vi "脉冲测试脚本.vi"(1 "参数":T1) -> (0 "Script":string)   [LabVIEW 2020]
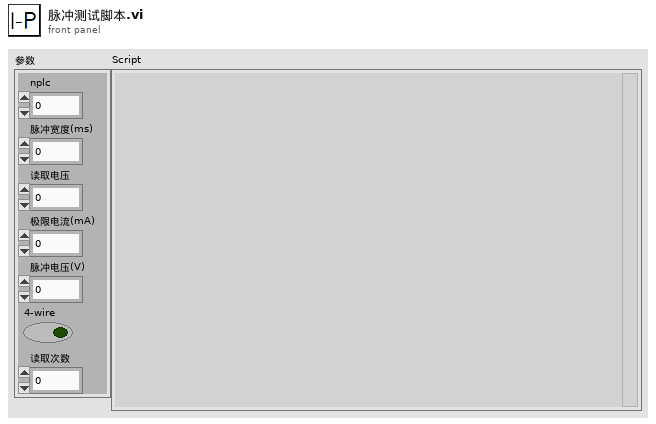
[diagram p1: front panel]
types:
  T1 = cluster{"nplc":dbl, "脉冲宽度(ms)":dbl, "读取电压":dbl, "极限电流(mA)":dbl, "脉冲电压(V)":dbl, "4-wire":bool, "读取次数":dbl}
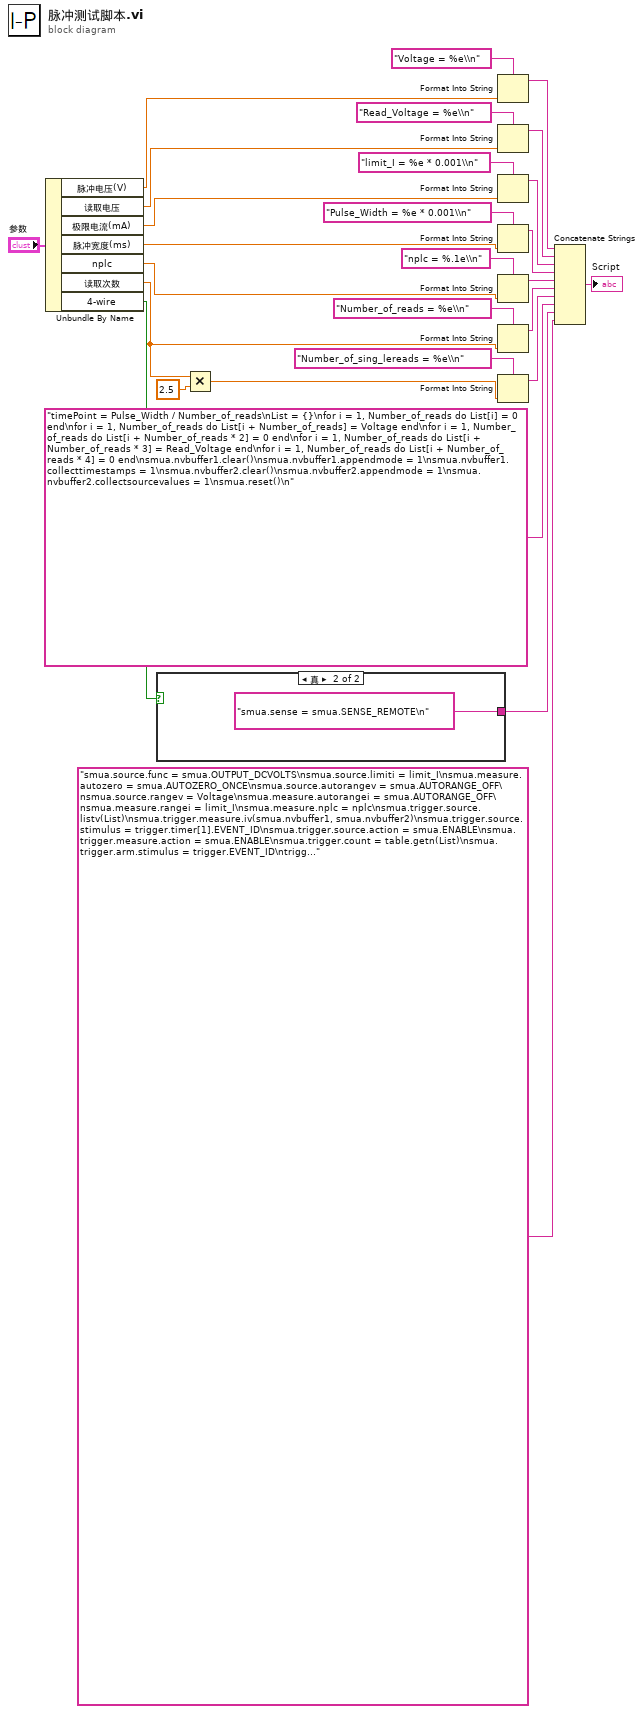
[diagram p0: block diagram]
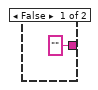
[diagram p2: hidden frame]
diagram:
  n1 = Unbundle By Name("参数") -> ("脉冲电压(V)"=w15:dbl, "读取电压"=w14:dbl, "极限电流(mA)"=w13:dbl, "脉冲宽度(ms)"=w12:dbl, "nplc"=w4:dbl, "读取次数"=w3:dbl, "4-wire"=w8:bool)
  n2 = case shown="真" w8 {
    tunnel: ["" "smua.sense = smua.SENSE_REMOTE\n"] -> w16
    frame False {
    }
    frame True {
    }
  }
  n3 = Multiply(x=w3, y=2.5) -> (x*y=w1:dbl)
  n4 = Format Into String(format string="Voltage = %e\\n" ("格式字符串"), w15) -> (resulting string=w25:string)  [unwired: 2 in, 1 out]
  n5 = Format Into String(format string="Read_Voltage = %e\\n" ("格式字符串"), w14) -> (resulting string=w23:string)  [unwired: 2 in, 1 out]
  n6 = Format Into String(format string="limit_I = %e * 0.001\\n" ("格式字符串"), w13) -> (resulting string=w22:string)  [unwired: 2 in, 1 out]
  n7 = Format Into String(format string="Pulse_Width = %e * 0.001\\n", w12) -> (resulting string=w20:string)  [unwired: 2 in, 1 out]
  n8 = Format Into String(format string="nplc = %.1e\\n", w4) -> (resulting string=w18:string)  [unwired: 2 in, 1 out]
  n9 = Format Into String(format string="Number_of_reads = %e\\n" ("格式字符串"), w3) -> (resulting string=w6:string)  [unwired: 2 in, 1 out]
  n10 = Format Into String(format string="Number_of_sing_lereads = %e\\n" ("格式字符串"), w1) -> (resulting string=w5:string)  [unwired: 2 in, 1 out]
  n11 = Concatenate Strings(w25, w23, w22, w20, w18, w6, w5, "timePoint = Pulse_Width / Number_of_reads\nList = {}\nfor i = 1, Number_of_reads do List[i] = 0 end\nfor i = 1, Number_of_reads do List[i + Number_of_reads] = Voltage end\nfor i = 1, Number_of_reads do List[i + Number_of_reads * 2] = 0 end\nfor i = 1, Number_of_reads do List[i + Number_of_reads * 3] = Read_Voltage end\nfor i = 1, Number_of_reads do List[i + Number_of_reads * 4] = 0 end\nsmua.nvbuffer1.clear()\nsmua.nvbuffer1.appendmode = 1\nsmua.nvbuffer1.collecttimestamps = 1\nsmua.nvbuffer2.clear()\nsmua.nvbuffer2.appendmode = 1\nsmua.nvbuffer2.collectsourcevalues = 1\nsmua.reset()\n", w16, "smua.source.func = smua.OUTPUT_DCVOLTS\nsmua.source.limiti = limit_I\nsmua.measure.autozero = smua.AUTOZERO_ONCE\nsmua.source.autorangev = smua.AUTORANGE_OFF\nsmua.source.rangev = Voltage\nsmua.measure.autorangei = smua.AUTORANGE_OFF\nsmua.measure.rangei = limit_I\nsmua.measure.nplc = nplc\nsmua.trigger.source.listv(List)\nsmua.trigger.measure.iv(smua.nvbuffer1, smua.nvbuffer2)\nsmua.trigger.source.stimulus = trigger.timer[1].EVENT_ID\nsmua.trigger.source.action = smua.ENABLE\nsmua.trigger.measure.action = smua.ENABLE\nsmua.trigger.count = table.getn(List)\nsmua.trigger.arm.stimulus = trigger.EVENT_ID\ntrigger.timer[1].reset()\ntrigger.timer[1].stimulus = smua.trigger.ARMED_EVENT_ID\ntrigger.timer[1].passthrough = false\ntrigger.timer[1].delay = timePoint\ntrigger.timer[1].count = table.getn(List)\nsmua.source.output = smua.OUTPUT_ON\nsmua.trigger.initiate()\ndelay(1e-3)\nsmua.trigger.arm.set()\nfunction _done()\n    Start = 1\n    Stop = Number_of_sing_lereads\n    repeat\n        if (bit.test(status.operation.instrument.smua.condition, 4) == false) then\n            smua.source.leveli = 0\n            smua.source.levelv = 0\n            smua.source.output = smua.OUTPUT_OFF\n            Stop = table.getn(List)\n            print(\"{\" .. Stop - Start + 1 .. \"}\")\n            printbuffer(Start, Stop, smua.nvbuffer1.timestamps)\n            printbuffer(Start, Stop, smua.nvbuffer2.sourcevalues)\n            printbuffer(Start, Stop, smua.nvbuffer1)\n            printbuffer(Start, Stop, smua.nvbuffer2)\n            print(\"{done}\")\n            return\n        elseif (smua.nvbuffer1.n > Stop) then\n            print(\"{\" .. Number_of_sing_lereads .. \"}\")\n            printbuffer(Start, Stop, smua.nvbuffer1.timestamps)\n            printbuffer(Start, Stop, smua.nvbuffer2.sourcevalues)\n            printbuffer(Start, Stop, smua.nvbuffer1)\n            printbuffer(Start, Stop, smua.nvbuffer2)\n            Start = Start + Number_of_sing_lereads\n            Stop = Stop + Number_of_sing_lereads\n        end\n        delay(timePoint)\n    until (false)\nend\n_done()\nreset()\n") -> (→"Script":string)
